vi "UP arjun kedua.vi"() -> ()   [LabVIEW 2021]
panel:
  in  "stop 4":bool
  in  "Free":bool
  in  "User":bool
  in  "Admin":bool
  in  "Ring":u16(ring) items=["Admin", "User", "Free"]
  in  "Delay":dbl(knob) scale=0.0..10.0
  out "c3":bool
  out "b3":bool
  out "d3":bool
  out "a3":bool
  out "g3":bool
  out "e3":bool
  out "f3":bool
  out "c2":bool
  out "b2":bool
  out "d2":bool
  out "a2":bool
  out "g2":bool
  out "e2":bool
  out "f2":bool
  out "c1":bool
  out "b1":bool
  out "d1":bool
  out "a1":bool
  out "g1":bool
  out "e1":bool
  out "f1":bool
  in  "Tab Control":enum32{"Page 1", "Page 2", "Page 3"}(tab)
  in  "Username":string
  in  "OK":bool
  in  "password":string
  in  "stop":bool
  in  "Ok 2":bool
  in  "Username 2":string
  in  "Password 2":string
  in  "stop 2":bool
  in  "stop 3":bool
  in  "Select":bool
  in  "switch":bool
  # "show"
  # "Fast"
  # "ADMIN"
  # "User"
  # "Username"
  # "Password"
  # "Free"
  # "Run"
  # "0 : ON\n1 : Acak"
  # "Clear"
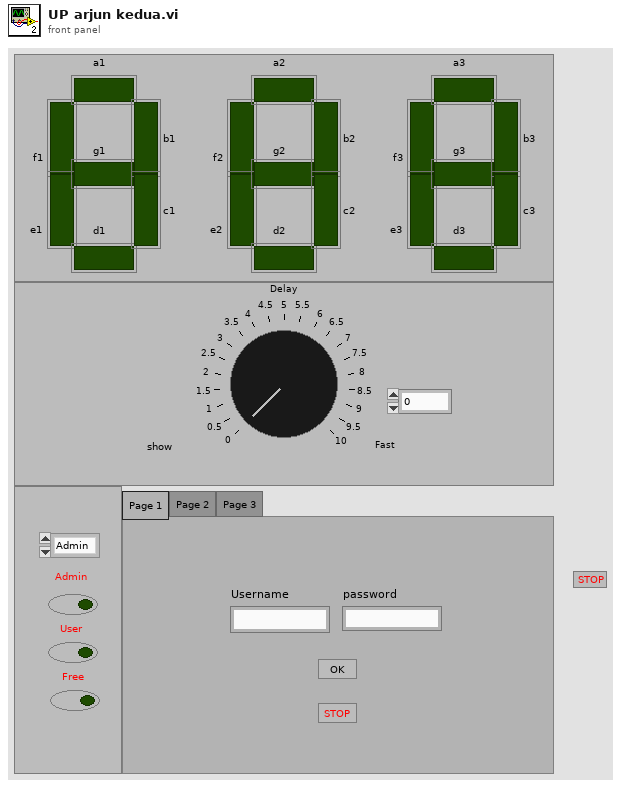
[diagram p1: front panel]
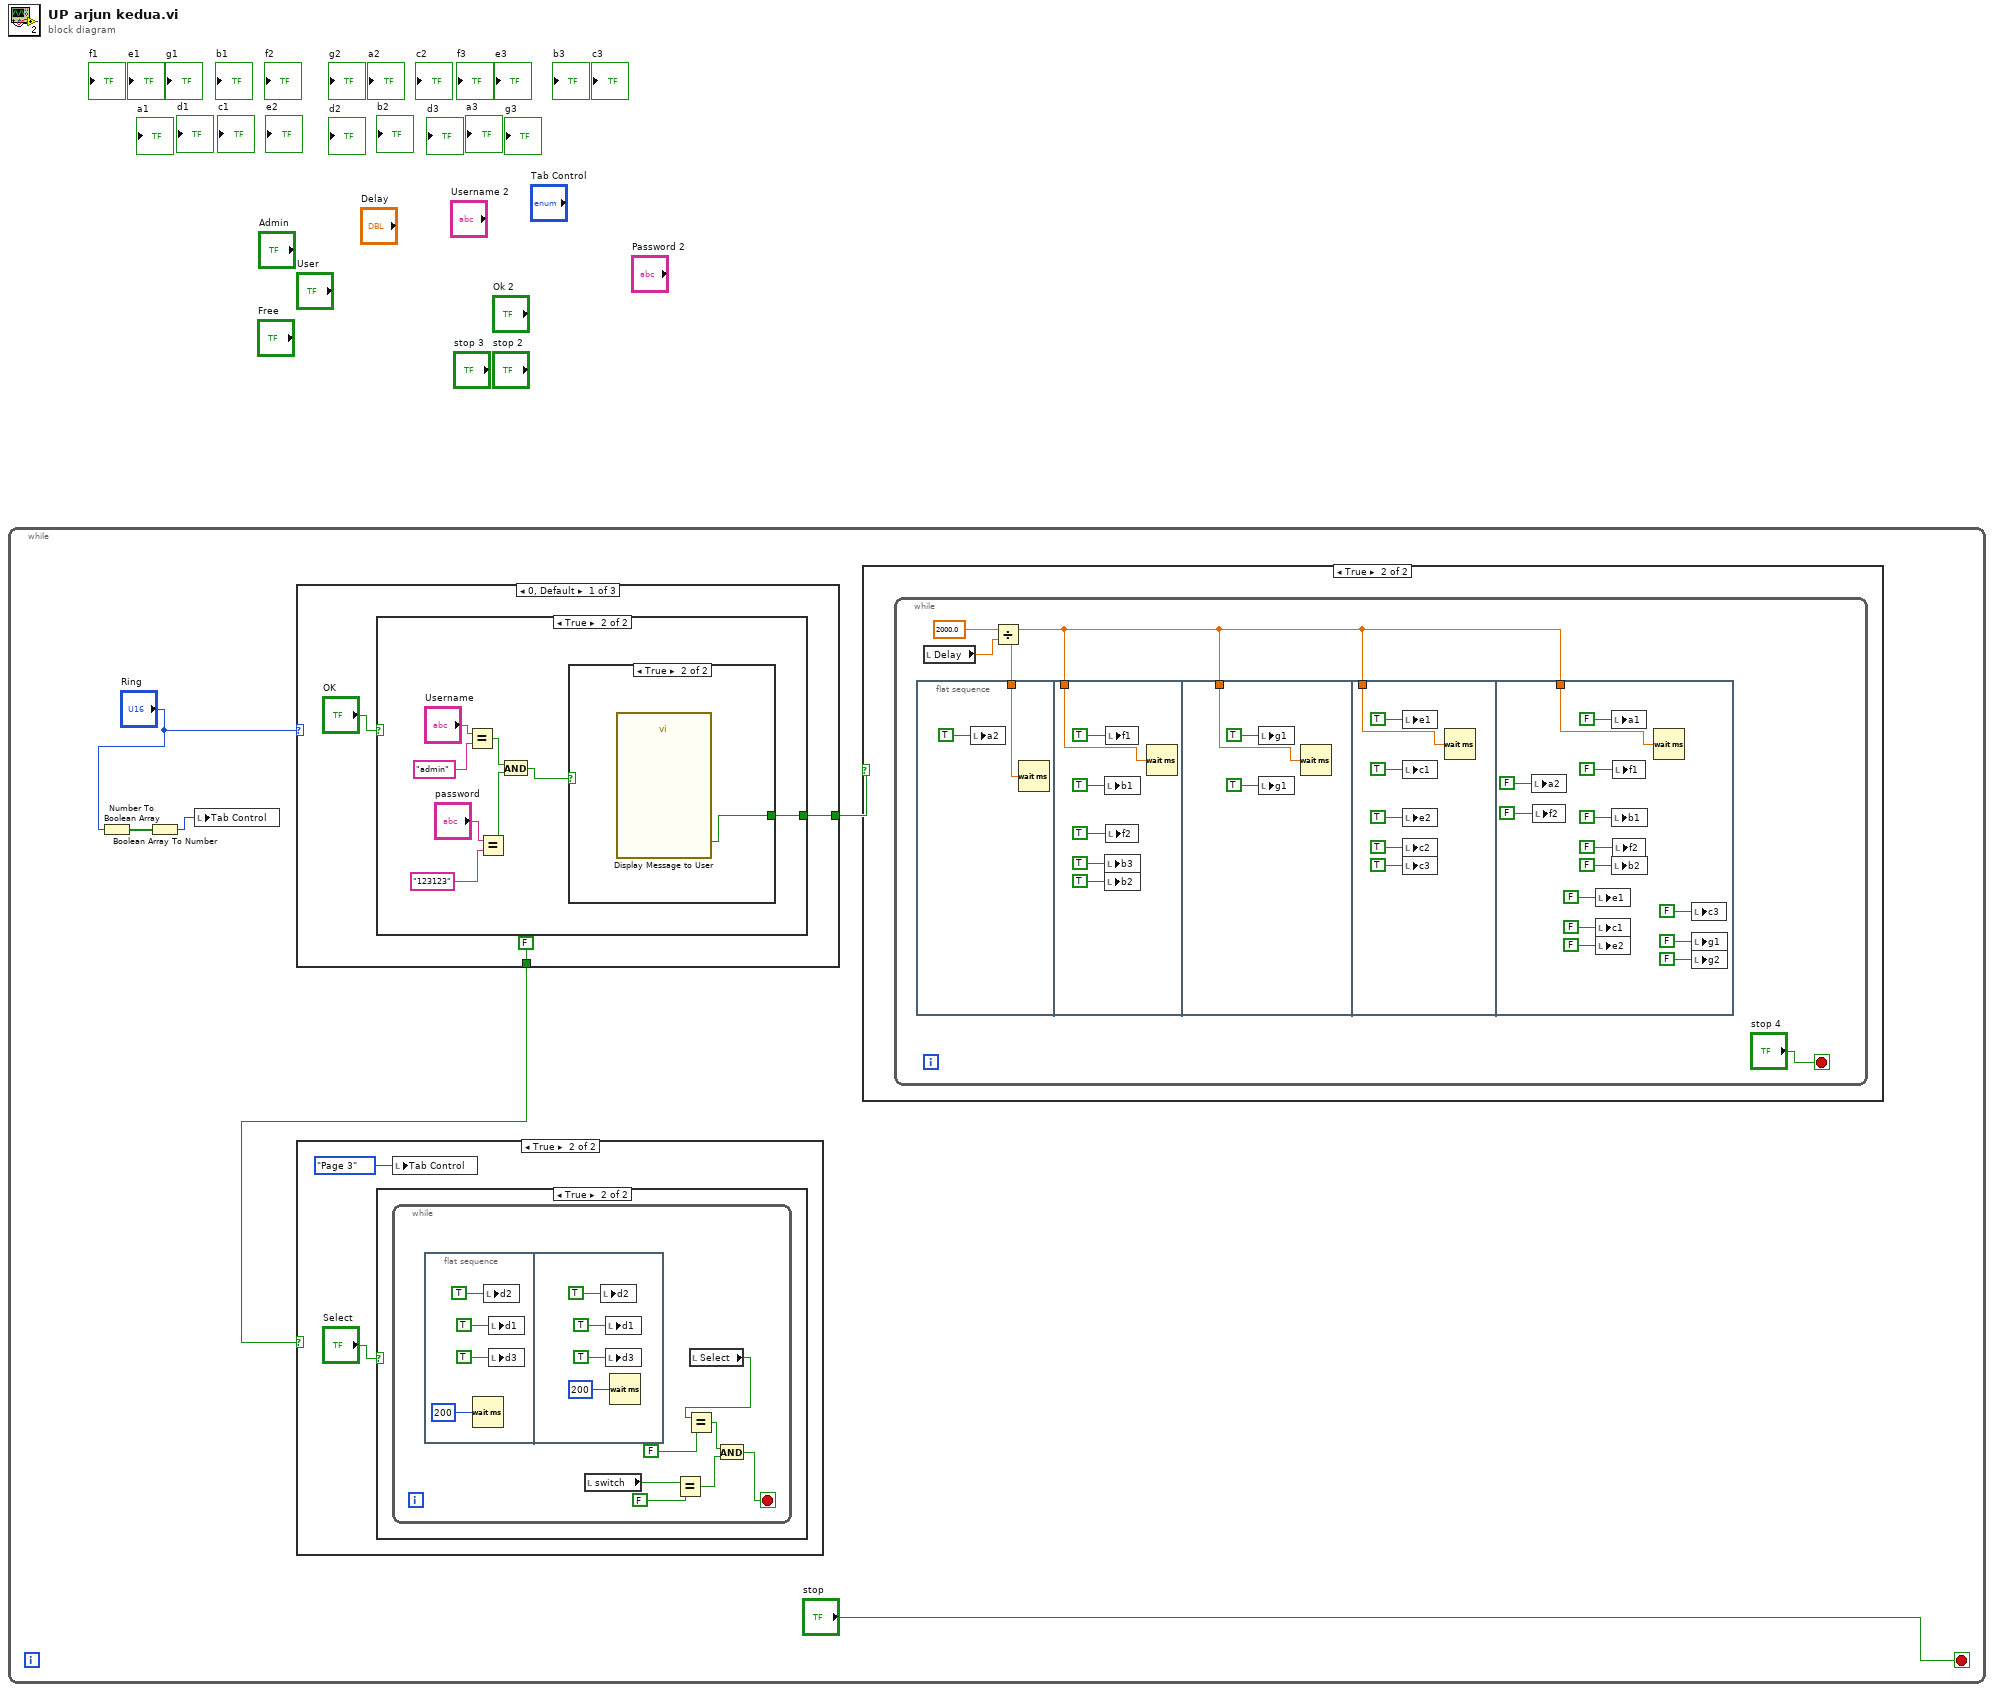
[diagram p0: block diagram]
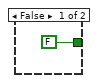
[diagram p5: hidden frame]
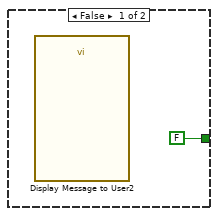
[diagram p6: hidden frame]
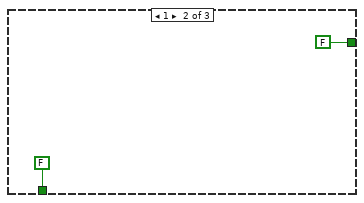
[diagram p7: hidden frame]
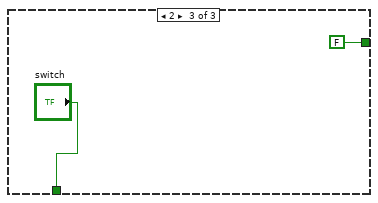
[diagram p8: hidden frame]
diagram:
  n1 = while {
    stop <- "stop" stop-if-true
    n2 = Number To Boolean Array(number="Ring") -> (Boolean array=w6:bool[])
    n3 = Boolean Array To Number(Boolean array=w6) -> (number=w4:u32)
    n4 = local write "Tab Control"(w4) -> ()
    n5 = case shown="0, Default" "Ring" {
      tunnel: [w60 FALSE FALSE] -> w3
      tunnel: [FALSE ("switch") FALSE ("switch") "switch"] -> w2
      frame 0, Default {
        n6 = case shown="True" "OK" {
          tunnel: [FALSE w64] -> w60
          frame False {
          }
          frame True {
            n7 = Equal?(x="Username", y="admin" ("Username")) -> (x = y?=w68:bool)
            n8 = Equal?(x="password", y="123123" ("password")) -> (x = y?=w63:bool)
            n9 = And(x=w68, y=w63) -> (x .and. y?=w67:bool)
            n10 = case shown="True" w67 {
              tunnel: [FALSE w72] -> w64
              frame False {
                n11 = call "Display Message to User2"() -> ()  [unwired: 10 in, 2 out]
              }
              frame True {
                n12 = call "Display Message to User"() -> ("OK"=w72:bool)  [unwired: 10 in, 1 out]
              }
            }
          }
        }
      }
      frame 1 {
      }
      frame 2 {
      }
    }
    n13 = case shown="True" w2 {
      frame False {
      }
      frame True {
        n14 = case shown="True" "Select" {
          frame False {
          }
          frame True {
            n15 = while {
              stop <- w13 stop-if-true
              n16 = flat-sequence {
                frame #0 {
                  n17 = Wait (ms)(milliseconds to wait=u32 200) -> ()  [unwired: 1 out]
                  n18 = local write "d2"(TRUE ("d2")) -> ()
                  n19 = local write "d1"(TRUE ("d2")) -> ()
                  n20 = local write "d3"(TRUE ("d2")) -> ()
                }
                frame #1 {
                  n21 = local write "d2"(TRUE ("d2")) -> ()
                  n22 = local write "d1"(TRUE ("d2")) -> ()
                  n23 = local write "d3"(TRUE ("d2")) -> ()
                  n24 = Wait (ms)(milliseconds to wait=u32 200) -> ()  [unwired: 1 out]
                }
              }
              n25 = local read "switch"() -> (w10:bool)
              n26 = Equal?(x=w10, y=FALSE) -> (x = y?=w15:bool)
              n27 = local read "Select"() -> (w12:bool)
              n28 = Equal?(x=w12, y=FALSE) -> (x = y?=w14:bool)
              n29 = And(x=w14, y=w15) -> (x .and. y?=w13:bool)
            }
          }
        }
        n30 = local write "Tab Control"(enum32{"Page 1", "Page 2", "Page 3"}."Page 3" ("Tab Control")) -> ()
      }
    }
    n31 = case shown="True" w3 {
      frame False {
      }
      frame True {
        n32 = while {
          stop <- "stop 4" stop-if-true
          n33 = flat-sequence {
            tunnel: w24 -> [w28]
            tunnel: w24 -> [w30]
            tunnel: w24 -> [w36]
            tunnel: w24 -> [w39]
            tunnel: w24 -> [w53]
            frame #0 {
              n34 = local write "a2"(TRUE ("d2")) -> ()
              n35 = Wait (ms)(milliseconds to wait=w28) -> ()  [unwired: 1 out]
            }
            frame #1 {
              n36 = local write "b1"(TRUE ("d2")) -> ()
              n37 = local write "b3"(TRUE ("d2")) -> ()
              n38 = local write "b2"(TRUE ("d2")) -> ()
              n39 = local write "f1"(TRUE ("d2")) -> ()
              n40 = local write "f2"(TRUE ("d2")) -> ()
              n41 = Wait (ms)(milliseconds to wait=w30) -> ()  [unwired: 1 out]
            }
            frame #2 {
              n42 = local write "g1"(TRUE ("d2")) -> ()
              n43 = local write "g1"(TRUE ("d2")) -> ()
              n44 = Wait (ms)(milliseconds to wait=w36) -> ()  [unwired: 1 out]
            }
            frame #3 {
              n45 = local write "e1"(TRUE ("d2")) -> ()
              n46 = local write "c1"(TRUE ("d2")) -> ()
              n47 = local write "e2"(TRUE ("d2")) -> ()
              n48 = local write "c2"(TRUE ("d2")) -> ()
              n49 = local write "c3"(TRUE ("d2")) -> ()
              n50 = Wait (ms)(milliseconds to wait=w39) -> ()  [unwired: 1 out]
            }
            frame #4 {
              n51 = local write "a2"(FALSE ("d2")) -> ()
              n52 = local write "f2"(FALSE ("d2")) -> ()
              n53 = local write "e1"(FALSE ("d2")) -> ()
              n54 = local write "c1"(FALSE ("d2")) -> ()
              n55 = local write "e2"(FALSE ("d2")) -> ()
              n56 = local write "a1"(FALSE ("d2")) -> ()
              n57 = local write "b1"(FALSE ("d2")) -> ()
              n58 = local write "b2"(FALSE ("d2")) -> ()
              n59 = local write "f1"(FALSE ("d2")) -> ()
              n60 = local write "f2"(FALSE ("d2")) -> ()
              n61 = Wait (ms)(milliseconds to wait=w53) -> ()  [unwired: 1 out]
              n62 = local write "c3"(FALSE ("d2")) -> ()
              n63 = local write "g1"(FALSE ("d2")) -> ()
              n64 = local write "g2"(FALSE ("d2")) -> ()
            }
          }
          n65 = local read "Delay"() -> (w26:dbl)
          n66 = Divide(x=2000.0, y=w26) -> (x/y=w24:dbl)
        }
      }
    }
  }
